vi "examplewhiledata_pass.vi"() -> ()   [LabVIEW 2020]
panel:
  out "index of elements":i32
  out "current i value":i32
  out "i value":i32
  out "element":i32
  out "size(s)":i32
  out "Array":i32[](array[numeric])
  out "Waveform Chart":cluster{i32, i32}(graph)
  out "XY Graph":cluster{i32[], i32[]}(graph)
  in  "stop":bool
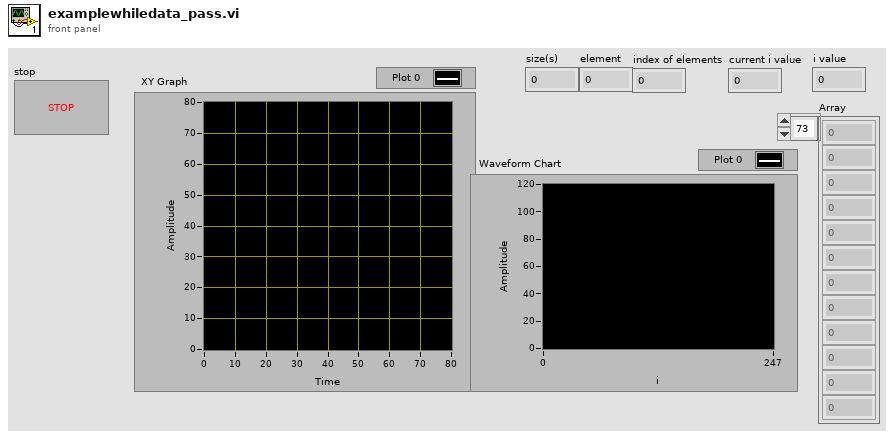
[diagram p1: front panel]
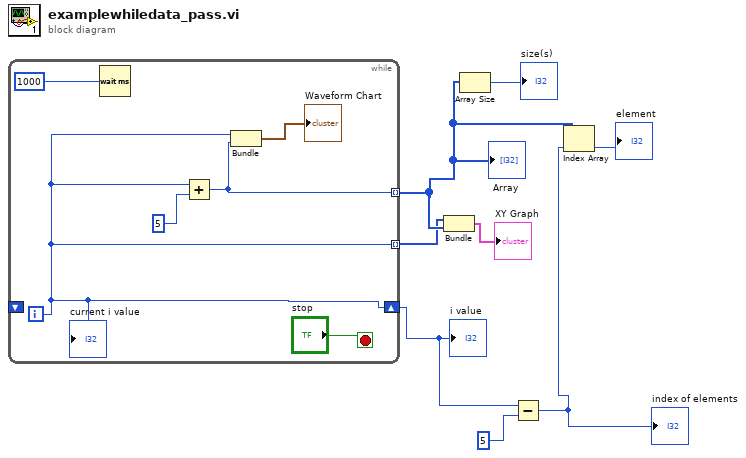
[diagram p0: block diagram]
diagram:
  n1 = while {
    tunnel: [w10] -> w5 mode=indexing
    tunnel: [w9] -> w4 mode=indexing
    shift-right: [w9] -> w2
    shift-left: _ -> [_]
    i -> [w9]
    stop <- "stop" stop-if-true
    n2 = Wait (ms)(milliseconds to wait=u32 1000) -> ()  [unwired: 1 out]
    n3 = Add(x=w9, y=5) -> (x+y=w10:i32)
    n4 = Bundle(w9, w10) -> (→"Waveform Chart":cluster{i32, i32})  [unwired: 1 in]
    "current i value" <- w9
  }
  "Array" <- w5
  "i value" <- w2
  n5 = Bundle(w4, w5) -> (→"XY Graph":cluster{i32[], i32[]})  [unwired: 1 in]
  n6 = Array Size(array=w5) -> (size(s)=→"size(s)":i32)
  n7 = Subtract(x=w2, y=5) -> (x-y=w1:i32)
  "index of elements" <- w1
  n8 = Index Array(array=w5, index=w1) -> (element=→"element":i32)
